vi "SetCursor.vi"   [LabVIEW 2019]
uses:
  <vilib>/Utility/cursorutil.llb/Set Cursor (Cursor ID).vi
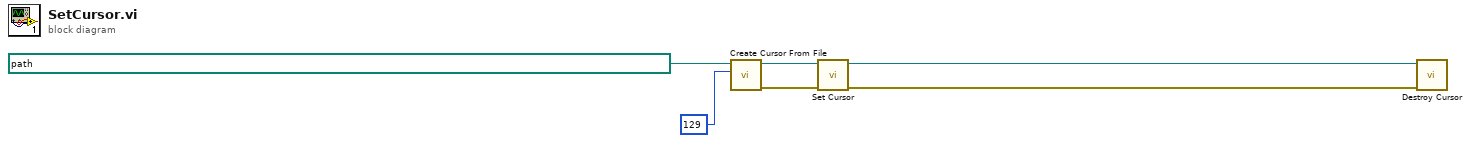
[diagram p0: block diagram]
diagram:
  n1 = call <vilib>:"Create Cursor From File.vi"("cursor resource ID"=i16 129, "cursor file"=path "D:/迅雷下载/windows_10_logo_cursors_by_alexgal23/Windows 10 Logo Cursors/Windows 10 Logo Black/NO.cur") -> ("error out"=w4:errorcluster, "cursor ID"=w3:refnum<k1>)  [unwired: 8 in]
  n2 = call-poly <vilib>:"Set Cursor.vi"("error in (no error)"=w4, "cursor ID"=w3) -> ("error out"=w1:errorcluster, "previous cursor ID"=w2:refnum<k1>)  [unwired: 8 in]
  n3 = call <vilib>:"Destroy Cursor.vi"("cursor ID"=w2, "error in (no error)"=w1) -> ()  [unwired: 8 in, 1 out]
